vi "Initialize-FilterWheel-SubVI.vi"(0 "Serial port":refnum<visa-resource-name>="COM1", 3 "error in":errorcluster) -> (7 "VISA resource name out":refnum<visa-resource-name>, 10 "error out":errorcluster)   [LabVIEW 2014]
uses:
  <vilib>/Instr/_visa.llb/VISA Configure Serial Port (Instr).vi
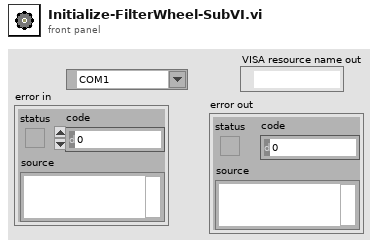
[diagram p1: front panel]
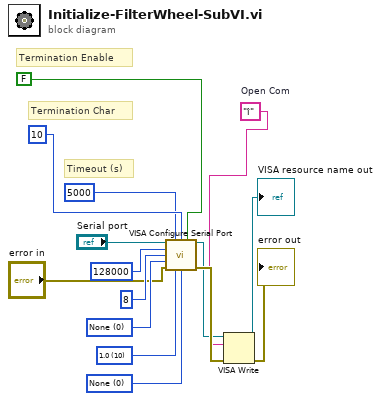
[diagram p0: block diagram]
diagram:
  w2 = "î"  # Open Com
  w7 = u16 0 items=["None"=0, "XON/XOFF"=1, "RTS/CTS"=2, "DTR/DSR"=4] ("flow control")
  w8 = u16 10 items=["1.0"=10, "1.5"=15, "2.0"=20] ("stop bits")
  w9 = u16 0 items=["None", "Odd", "Even", "Mark", "Space"] ("parity")
  # "Termination Char"
  # "Termination Enable"
  # "Timeout (s)"
  n1 = call-poly "VISA Configure Serial Port"("VISA resource name"="Serial port", "timeout (10sec)"=u32 5000 ("timeout (ms)"), "termination char\n(0xA = '\\n' = LF)"=u8 10 ("termination char\n(0xA = '\\n' = LF)"), "Enable Termination\nChar (T)"=FALSE ("End read on termination character?"), "baud rate (9600)"=u32 128000 ("timeout (ms)"), "data bits (8)"=u16 8 ("data bits"), "parity (0:none)"=w9, "error in (no error)"="error in", "stop bits (10: 1 bit)"=w8, "flow control (0:none)"=w7) -> ("VISA resource name out"=w5:refnum<visa-resource-name>, "error out"=w6:errorcluster)  [unwired: 4 in]
  n2 = VISA Write(VISA resource name=w5, write buffer=w2, error in (no error)=w6) -> (VISA resource name out=→"VISA resource name out":refnum<visa-resource-name>, error out=→"error out":errorcluster)  [unwired: 1 out]
